vi "Build Async Send Method.vi"(6 "Wiring Spec":T2, 7 "Async AF Library FQN":string, 8 "error in (no error)":errorcluster, 9 "AF Library FQN":string, 10 "References":T1, 11 "Send VI":refnum<vi>) -> (0 "error out":errorcluster)   [LabVIEW 2023, in "Message Maker.lvclass"]
doc: "Build The send vi for the new Async message"
uses:
  Message Maker.lvclass
  Wiring Spec.ctl
  Connector Pane Position.ctl
  Scripting Refs.ctl
  <vilib>/Utility/traverseref.llb/TRef TravTarget.ctl
  <vilib>/Utility/miscctls.llb/LVPointTypeDef.ctl
  Message Maker.lvclass/Message Maker.ctl
  <vilib>/Utility/traverseref.llb/VI Scripting - Traverse.lvlib
  <vilib>/LabVIEW Icon API/LabVIEW Icon API.lvlib
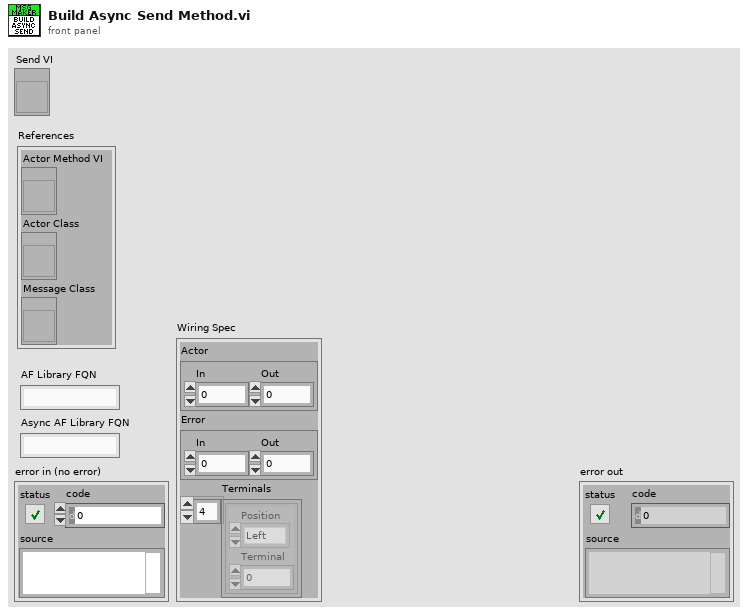
[diagram p1: front panel]
types:
  T1 = typedef "Message Maker.lvclass/Scripting Refs.ctl" = cluster{"Actor Method VI":refnum<vi>, "Actor Class":refnum<vi>, "Message Class":refnum<vi>}
  T2 = typedef "Message Maker.lvclass/Wiring Spec.ctl" = cluster{"Actor":cluster{"In":i32, "Out":i32}, "Error":cluster{"In":i32, "Out":i32}, "Terminals":cluster{"Position":T3, "Terminal":i32}[]}
  T3 = typedef "Message Maker.lvclass/Connector Pane Position.ctl" = enum16{"Left", "Top", "Bottom", "Right"}
  T4 = cluster{"Left":cluster{"Position":i16, "Index":i32}[], "Bottom":cluster{"Position":i16, "Index":i32}[], "Right":cluster{"Position":i16, "Index":i32}[], "Top":cluster{"Position":i16, "Index":i32}[]}
  T5 = enum16{"Replace Classes", "Configure Connector", "Add FP Controls", "Wire Bundle", "Wire Unbundle", "Wire Property Node", "Set Icon and Desc", "Build BD"}
  T6 = typedef "TRef TravTarget.ctl" = enum16{"FP", "BD", "Other"}
  T7 = typedef "LVPointTypeDef.ctl" = cluster{"Horizontal":i16, "Vertical":i16}
  T8 = typedef "LVRectTypeDef.ctl" = cluster{"Left":i16, "Top":i16, "Right":i16, "Bottom":i16}
  T9 = enum16{"Invalid Wire Rule", "Required", "Recommended", "Optional", "Dynamic Dispatch"}[]
  T10 = cluster{cluster{"Position":i16, "Index":i32}[]}[]
  T11 = enum16{"Invalid Wire Rule", "Required", "Recommended", "Optional", "Dynamic Dispatch"}
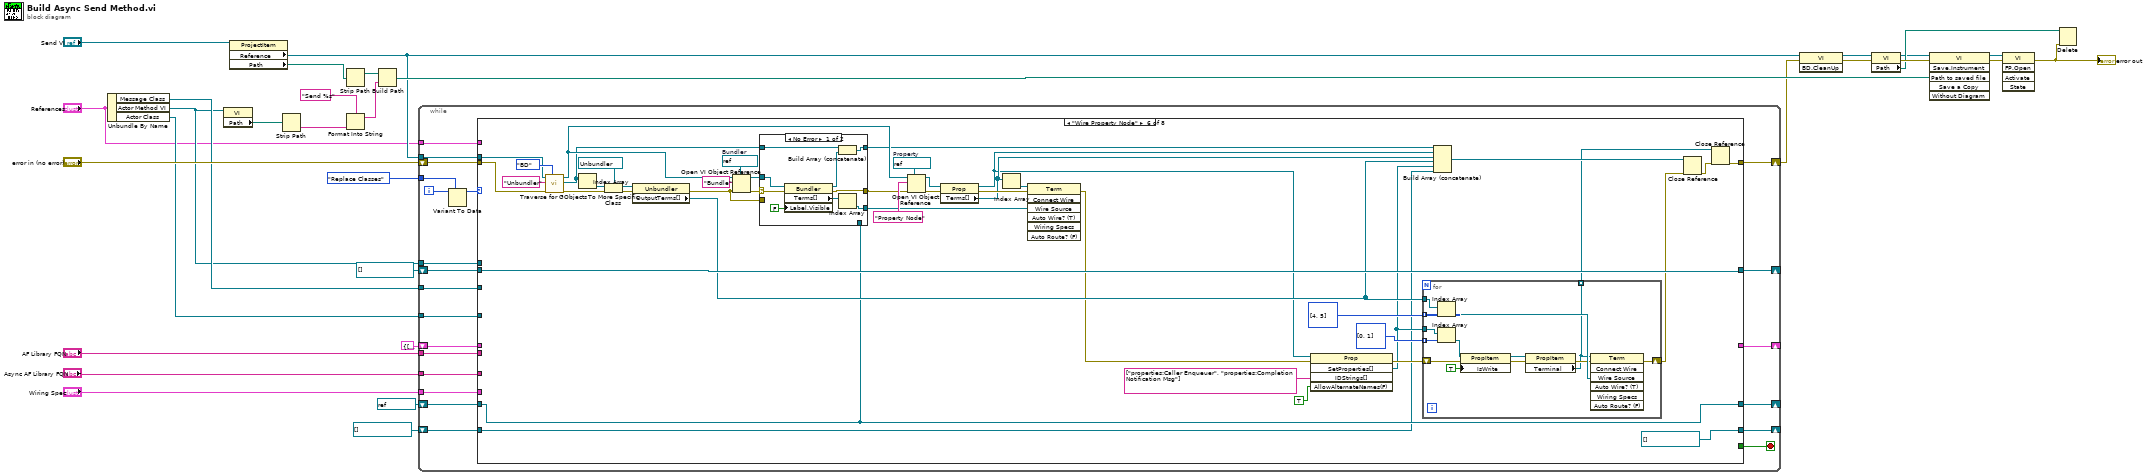
[diagram p0: block diagram]
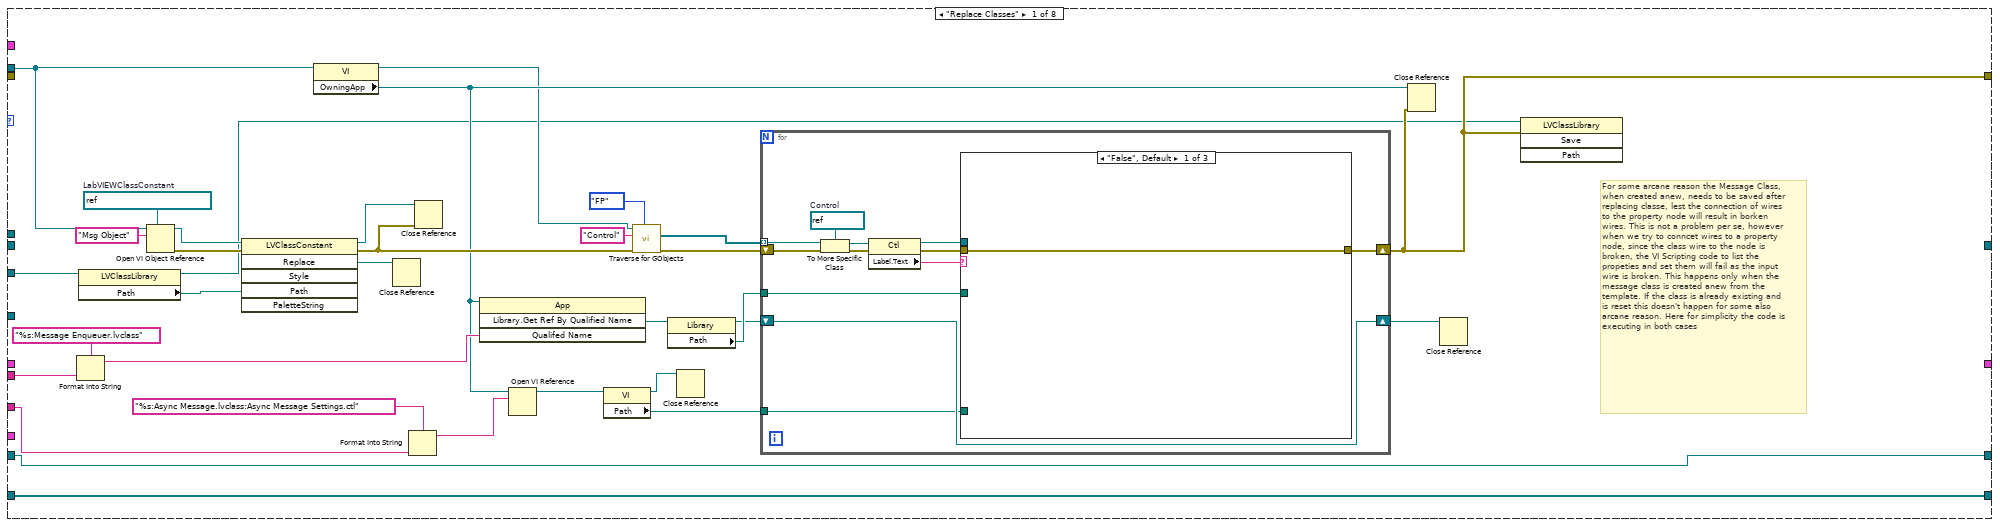
[diagram p2: hidden frame]
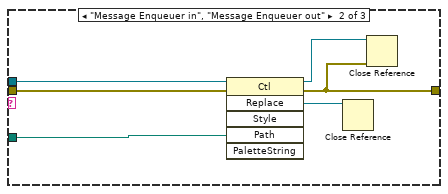
[diagram p3: hidden frame]
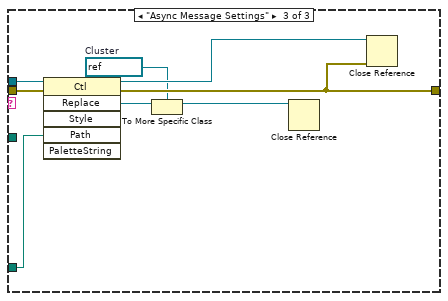
[diagram p4: hidden frame]
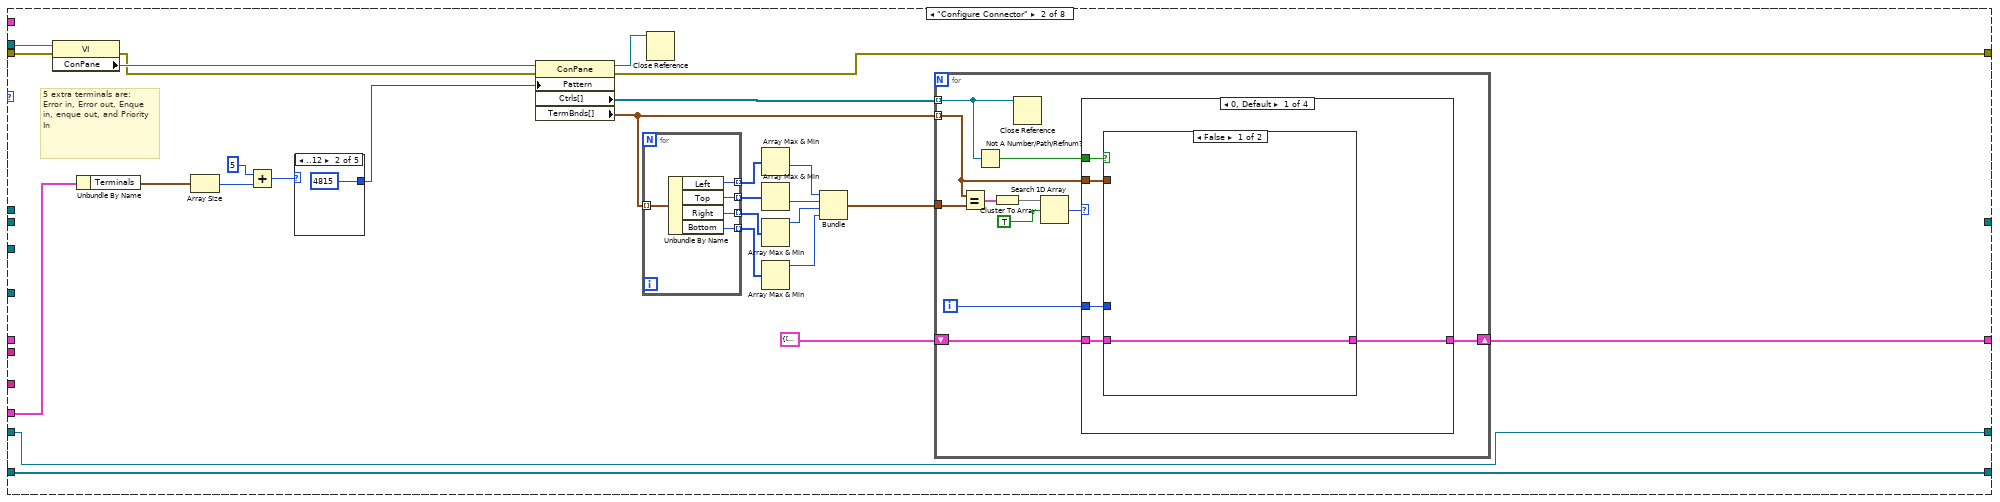
[diagram p5: hidden frame]
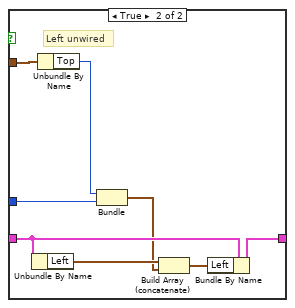
[diagram p6: hidden frame]
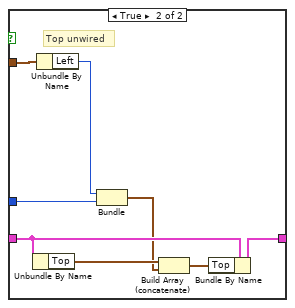
[diagram p8: hidden frame]
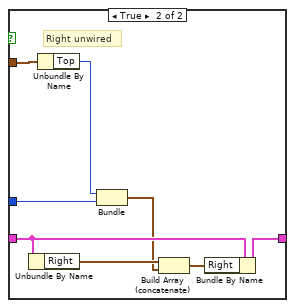
[diagram p10: hidden frame]
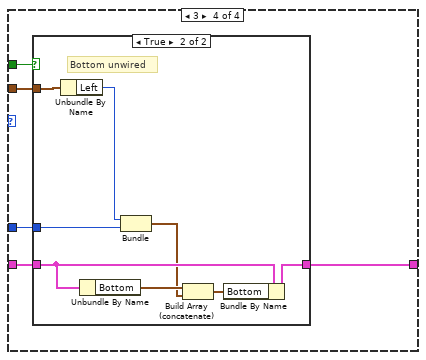
[diagram p11: hidden frame]
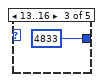
[diagram p14: hidden frame]
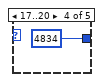
[diagram p15: hidden frame]
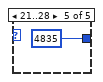
[diagram p16: hidden frame]
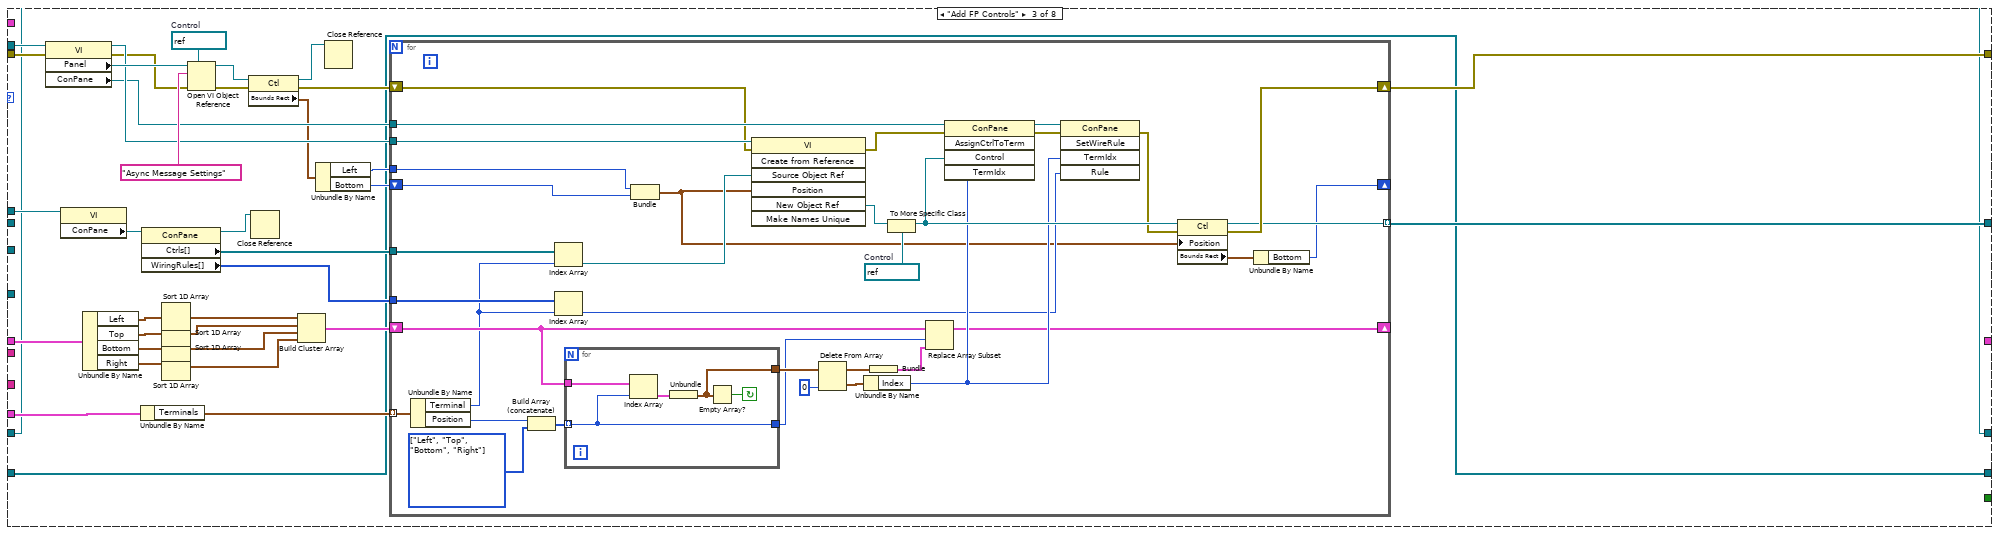
[diagram p17: hidden frame]
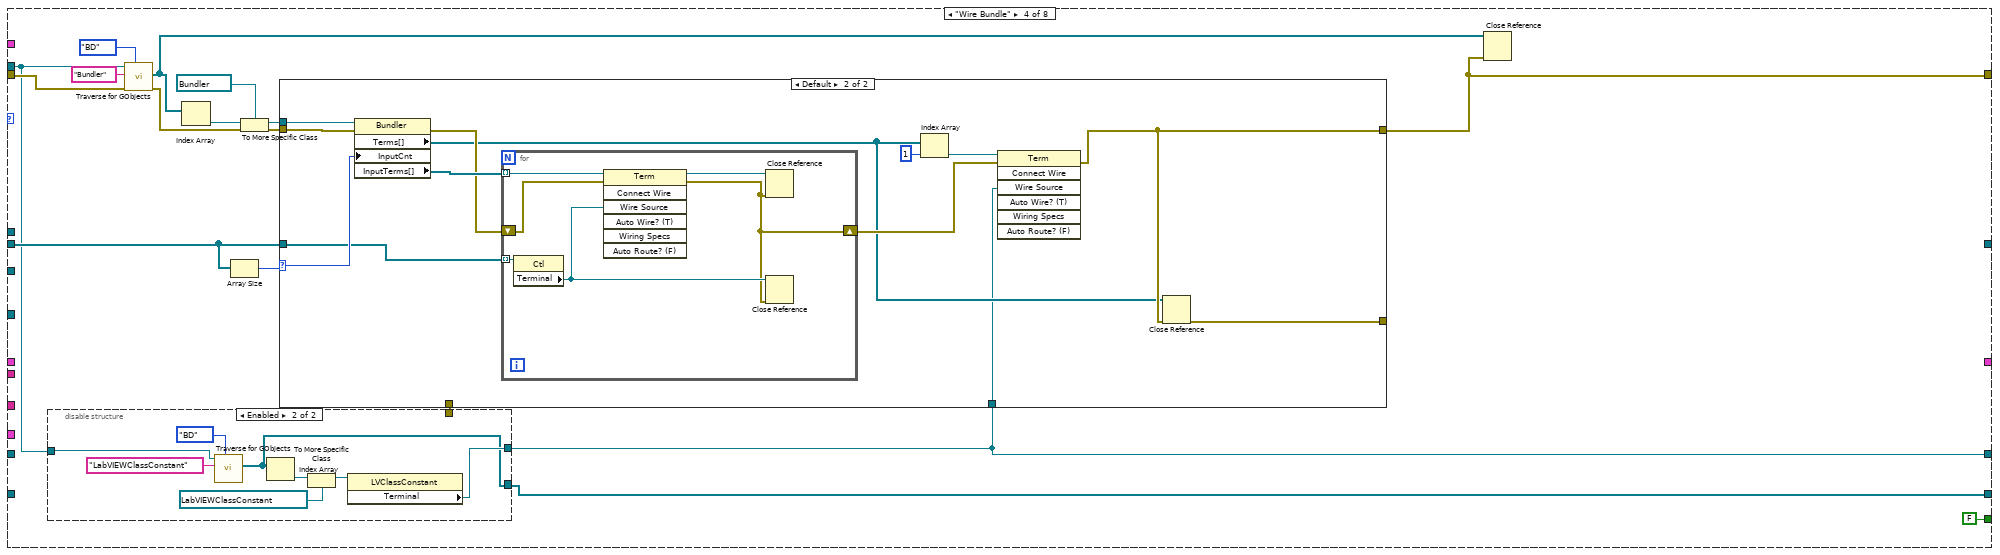
[diagram p18: hidden frame]
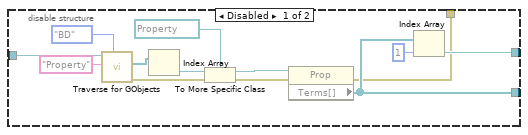
[diagram p19: hidden frame]
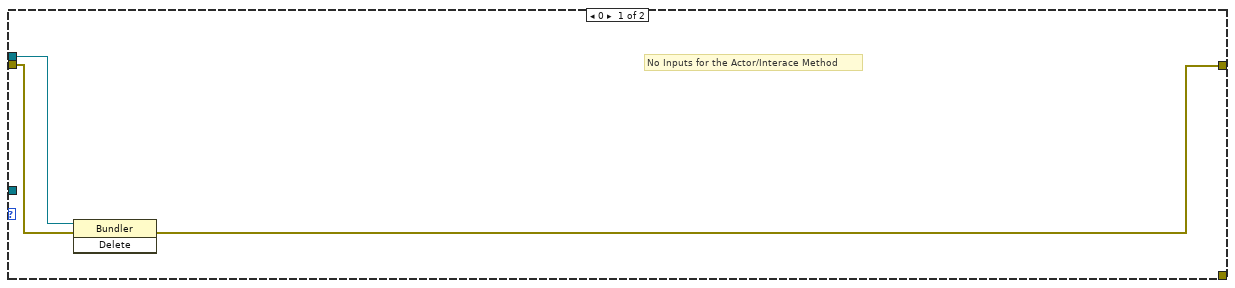
[diagram p20: hidden frame]
diagram:
  n1 = Unbundle By Name("References") -> ("Message Class"=w14:refnum<vi>, "Actor Method VI"=w9:refnum<vi>, "Actor Class"=w13:refnum<vi>)
  n2 = property class="VI"(reference=w9) -> ("Path"=w8:path)  [unwired: 1 in, 2 out]
  n3 = property class="ProjectItem"(reference="Send VI") -> ("Reference"=w22:refnum<vi>, "Path"=w28:path)  [unwired: 1 in, 2 out]
  n4 = Strip Path(path=w8) -> (name=w7:string)  [unwired: 1 out]
  n5 = Strip Path(path=w28) -> (stripped path=w27:path)  [unwired: 1 out]
  n6 = Format Into String(format string="Send %s", w7) -> (resulting string=w26:string)  [unwired: 2 in, 1 out]
  n7 = Build Path(base path=w27, name or relative path=w26) -> (appended path=w25:path)
  n8 = while {
    tunnel: T5."Replace Classes" -> [w53]
    tunnel: "Wiring Spec" -> [w50]
    tunnel: w22 -> [w49]
    tunnel: w9 -> [w48]
    shift-right: [w45] -> w20
    shift-left: "error in (no error)" -> [w46]
    shift-right: [w44] -> _
    shift-left: T4 {"Left"=[], "Bottom"=[], "Right"=[], "Top"=[]} -> [w43]
    shift-right: [w42] -> _
    shift-left: refnum<vi>[] [] -> [w41]
    tunnel: w14 -> [w40]
    tunnel: w13 -> [w39]
    tunnel: "AF Library FQN" -> [w38]
    shift-right: [w37] -> _
    shift-left: refnum<vi>[] [] ("Terms[]") -> [w36]
    tunnel: "Async AF Library FQN" -> [w35]
    tunnel: "References" -> [w34]
    shift-right: [w33] -> _
    shift-left: refnum<vi> refnum ("Terminal") -> [w32]
    i -> [w52]
    stop <- w47 stop-if-true
    n9 = Variant To Data(type=w53, Variant=w52) -> (data=w51:T5)  [unwired: 1 in, 1 out]
    n10 = case shown="\"Wire Property Node\"" w51 {
      tunnel: w50 -> [_ w140 w243 _ _ _ _ _]
      tunnel: w49 -> [w76 w139 w252 w297 w368 w413 w469 w493]
      tunnel: w48 -> [_ _ w245 _ _ _ w470 _]
      tunnel: [_ _ _ FALSE FALSE _ _ TRUE] -> w47
      tunnel: w46 -> [_ w134 w238 w309 w379 w414 w453 w479]
      tunnel: [w56 w132 w235 w298 w370 w422 w451 w487] -> w45
      tunnel: [_ w116 _ _ _ _ _ _] -> w44
      tunnel: w43 -> [_ _ w234 _ _ _ _ _]
      tunnel: [_ _ w222 _ w360 w412 _ _] -> w42
      tunnel: w41 -> [_ _ _ w304 w360 w412 _ _]
      tunnel: w40 -> [w84 _ _ _ _ _ w462 _]
      tunnel: w39 -> [_ _ _ _ _ _ w460 _]
      tunnel: w38 -> [w60 _ _ _ _ _ _ _]
      tunnel: [w62 w115 w218 w296 w363 refnum<vi>[] [] ("References") w450 w516] -> w37
      tunnel: w36 -> [w62 w115 w218 _ w363 w383 w450 w516]
      tunnel: w35 -> [w59 _ _ _ _ _ _ w475]
      tunnel: w34 -> [_ _ _ _ _ _ _ _]
      tunnel: [w54 w114 w217 w293 w353 w384 w449 w471] -> w33
      tunnel: w32 -> [w54 w114 w217 _ w353 w384 w449 w471]
      frame "Replace Classes" {
        w82 = refnum<vi> refnum  # LabVIEWClassConstant
        # "For some arcane reason the Message Class, when created anew, needs to be saved after replacing classe, lest the connection of wires to the property node will result in borken wires. This is not a problem per se, however when we try to conncet wires to a property node, since the class wire to the node is broken, the VI Scripting code to list the propeties and set them will fail as the input wire is broken. This happens only when the message class is created anew from the template. If the class is already existing and is reset this doesn't happen for some also arcane reason. Here for simplicity the code is executing in both cases"
        n11 = Format Into String(format string="%s:Message Enqueuer.lvclass", w60) -> (resulting string=w65:string)  [unwired: 2 in, 1 out]
        n12 = property class="LVClassLibrary"(reference=w84) -> (reference out=w55:refnum<vi>, "Path"=w86:path)  [unwired: 1 in, 1 out]
        n13 = Open VI Object Reference(7:w82, 10:"Msg Object" ("name/order"), 11:w76) -> (0:w83:errorcluster, 3:w58:refnum<vi>)  [unwired: 1 in]
        n14 = invoke class="LVClassConstant" method="Replace"(reference=w58, error in=w83, "Path"=w86) -> (reference out=w81:refnum<vi>, error out=w77:errorcluster, "Replace"=w85:refnum<vi>)  [unwired: 3 in, 3 out]
        n15 = property class="VI"(reference=w76) -> (reference out=w57:refnum<vi>, "OwningApp"=w63:refnum<vi>)  [unwired: 1 in, 1 out]
        n16 = Close Reference(reference=w85) -> ()  [unwired: 1 in, 1 out]
        n17 = Format Into String(format string="%s:Async Message.lvclass:Async Message Settings.ctl", w59) -> (resulting string=w69:string)  [unwired: 2 in, 1 out]
        n18 = Close Reference(reference=w81, error in (no error)=w77) -> ()  [unwired: 1 out]
        n19 = invoke class="App" method="Library.Get Ref By Qualified Name"(reference=w63, "Qualifed Name"=w65) -> ("Library.Get Ref By Qualified Name"=w73:refnum<vi>)  [unwired: 2 in, 3 out]
        n20 = Open VI Reference(application reference (local)=w63, vi path=w69) -> (vi reference=w68:refnum<vi>)  [unwired: 4 in, 1 out]
        n21 = property class="VI"(reference=w68) -> (reference out=w64:refnum<vi>, "Path"=w67:path)  [unwired: 1 in, 1 out]
        n22 = call <vilib>:"Traverse for GObjects.vi"("Traverse Target"=TRef_TravTarget."FP", "error in (no error)"=w77, "Class Name"="Control" ("name/order"), "VI Refnum"=w57) -> ("error out"=w78:errorcluster, "References"=w74:refnum<vi>[])  [unwired: 4 in, 2 out]
        n23 = property class="Library"(reference=w73) -> (reference out=w71:refnum<vi>, "Path"=w72:path)  [unwired: 1 in, 1 out]
        n24 = Close Reference(reference=w64) -> ()  [unwired: 1 in, 1 out]
        n25 = for {
          tunnel: w74 -> [w91] mode=indexing
          tunnel: w72 -> [w97]
          shift-right: [w96] -> w56
          shift-left: w78 -> [w98]
          shift-right: [w95] -> w70
          shift-left: w71 -> [w95]
          tunnel: w67 -> [w87]
          w89 = refnum<vi> refnum  # Control
          n26 = To More Specific Class(target class=w89, reference=w91, error in=w98) -> (specific class reference=w90:refnum<vi>, error out=w92:errorcluster)
          n27 = property class="Ctl"(reference=w90, error in=w92) -> (reference out=w93:refnum<vi>, error out=w94:errorcluster, "Label.Text"=w88:string)
          n28 = case shown="\"False\", Default" w88 {
            tunnel: w97 -> [_ w103 _]
            tunnel: [w99 w102 w111] -> w96
            tunnel: w94 -> [w99 w101 w110]
            tunnel: w93 -> [_ w100 w109]
            tunnel: w87 -> [_ _ w108]
            frame "False", Default {
            }
            frame "Message Enqueuer in", "Message Enqueuer out" {
              n29 = invoke class="Ctl" method="Replace"(reference=w100, error in=w101, "Path"=w103) -> (reference out=w105:refnum<vi>, error out=w102:errorcluster, "Replace"=w104:refnum<vi>)  [unwired: 3 in, 3 out]
              n30 = Close Reference(reference=w104) -> ()  [unwired: 1 in, 1 out]
              n31 = Close Reference(reference=w105, error in (no error)=w102) -> ()  [unwired: 1 out]
            }
            frame "Async Message Settings" {
              w106 = refnum<vi> refnum  # Cluster
              n32 = invoke class="Ctl" method="Replace"(reference=w109, error in=w110, "Path"=w108) -> (reference out=w113:refnum<vi>, error out=w111:errorcluster, "Replace"=w112:refnum<vi>)  [unwired: 3 in, 3 out]
              n33 = To More Specific Class(target class=w106, reference=w112) -> (specific class reference=w107:refnum<vi>)  [unwired: 1 in, 1 out]
              n34 = Close Reference(reference=w107) -> ()  [unwired: 1 in, 1 out]
              n35 = Close Reference(reference=w113, error in (no error)=w111) -> ()  [unwired: 1 out]
            }
          }
        }
        n36 = Close Reference(reference=w63, error in (no error)=w56) -> ()  [unwired: 1 out]
        n37 = Close Reference(reference=w70) -> ()  [unwired: 1 in, 1 out]
        n38 = invoke class="LVClassLibrary" method="Save"(reference=w55, error in=w56) -> ()  [unwired: 2 in, 4 out]
      }
      frame "Configure Connector" {
        # "5 extra terminals are:\nError in, Error out, Enque in, enque out, and Priority In"
        n39 = property class="VI"(reference=w139, error in=w134) -> (error out=w133:errorcluster, "ConPane"=w138:refnum<vi>)  [unwired: 1 out]
        n40 = Unbundle By Name(w140) -> ("Terminals"=w137:cluster{"Position":T3, "Terminal":i32}[])
        n41 = Array Size(array=w137) -> (size(s)=w131:i32)
        n42 = Add(x=5, y=w131) -> (x+y=w129:i32)
        n43 = case shown="..12" w129 {
          tunnel: [_ u32 4815 ("Pattern") u32 4833 ("Pattern") u32 4834 ("Pattern") u32 4835 ("Pattern")] -> w135
          frame Default {
          }
          frame ..12 {
          }
          frame 13..16 {
          }
          frame 17..20 {
          }
          frame 21..28 {
          }
        }
        n44 = property class="ConPane"(reference=w138, error in=w133, "Pattern"=w135) -> (reference out=w136:refnum<vi>, error out=w132:errorcluster, "Ctrls[]"=w122:refnum<vi>[], "TermBnds[]"=w120:T8[])
        n45 = for {
          tunnel: w120 -> [w212] mode=indexing
          tunnel: [w211] -> w128 mode=indexing
          tunnel: [w210] -> w127 mode=indexing
          tunnel: [w209] -> w126 mode=indexing
          tunnel: [w208] -> w125 mode=indexing
          n46 = Unbundle By Name(w212) -> ("Left"=w211:i16, "Top"=w210:i16, "Right"=w209:i16, "Bottom"=w208:i16)
        }
        n47 = Close Reference(reference=w136) -> ()  [unwired: 1 in, 1 out]
        n48 = Array Max & Min(array=w128) -> (min value=w119:i16)  [unwired: 3 out]
        n49 = Array Max & Min(array=w127) -> (min value=w118:i16)  [unwired: 3 out]
        n50 = Array Max & Min(array=w126) -> (max value=w124:i16)  [unwired: 3 out]
        n51 = Array Max & Min(array=w125) -> (max value=w123:i16)  [unwired: 3 out]
        n52 = Bundle(w119, w118, w124, w123) -> (w121:cluster{i16, i16, i16, i16})  [unwired: 1 in]
        n53 = for {
          tunnel: w122 -> [w146] mode=indexing
          tunnel: w121 -> [w151]
          tunnel: w120 -> [w143] mode=indexing
          shift-right: [w142] -> w116
          shift-left: T4 {"Left"=[], "Bottom"=[], "Right"=[], "Top"=[]} -> [w144]
          i -> [w141]
          n54 = Equal?(x=w143, y=w151) -> (x = y?=w150:cluster{bool, bool, bool, bool})
          n55 = Not A Number/Path/Refnum?(number/path/refnum=w146) -> (NaN/Path/Refnum?=w145:bool)
          n56 = Cluster To Array(cluster=w150) -> (array=w149:bool[])
          n57 = Close Reference(reference=w146) -> ()  [unwired: 1 in, 1 out]
          n58 = Search 1D Array(1D array=w149, element=TRUE) -> (index of element=w147:i32)  [unwired: 1 in]
          n59 = case shown="0, Default" w147 {
            tunnel: w145 -> [w156 w170 w184 w198]
            tunnel: w144 -> [w155 w169 w183 w197]
            tunnel: w143 -> [w154 w168 w182 w196]
            tunnel: [w153 w167 w181 w195] -> w142
            tunnel: w141 -> [w152 w166 w180 w194]
            frame 0, Default {
              n60 = case shown="False" w156 {
                tunnel: w155 -> [w157 w164]
                tunnel: w154 -> [_ w165]
                tunnel: [w157 w161] -> w153
                tunnel: w152 -> [_ w162]
                frame False {
                }
                frame True {
                  # "Left unwired"
                  n61 = Unbundle By Name(w164) -> ("Left"=w160:cluster{"Position":i16, "Index":i32}[])
                  n62 = Unbundle By Name(w165) -> ("Top"=w163:i16)
                  n63 = Bundle("Top"=w163, w162) -> (w158:cluster{"Top":i16, i32})  [unwired: 1 in]
                  n64 = Build Array (concatenate)(w160, w158) -> (w159:cluster{"Top":i16, "Index":i32}[])
                  n65 = Bundle By Name(cluster=w164, "Left"=w159) -> (w161:T4)
                }
              }
            }
            frame 1 {
              n66 = case shown="False" w170 {
                tunnel: w169 -> [w171 w178]
                tunnel: w168 -> [_ w179]
                tunnel: [w171 w175] -> w167
                tunnel: w166 -> [_ w176]
                frame False {
                }
                frame True {
                  # "Top unwired"
                  n67 = Unbundle By Name(w178) -> ("Top"=w174:cluster{"Position":i16, "Index":i32}[])
                  n68 = Unbundle By Name(w179) -> ("Left"=w177:i16)
                  n69 = Bundle("Left"=w177, w176) -> (w172:cluster{"Left":i16, i32})  [unwired: 1 in]
                  n70 = Build Array (concatenate)(w174, w172) -> (w173:cluster{"Left":i16, "Index":i32}[])
                  n71 = Bundle By Name(cluster=w178, "Top"=w173) -> (w175:T4)
                }
              }
            }
            frame 2 {
              n72 = case shown="False" w184 {
                tunnel: w183 -> [w185 w192]
                tunnel: w182 -> [_ w193]
                tunnel: [w185 w189] -> w181
                tunnel: w180 -> [_ w190]
                frame False {
                }
                frame True {
                  # "Right unwired"
                  n73 = Unbundle By Name(w192) -> ("Right"=w188:cluster{"Position":i16, "Index":i32}[])
                  n74 = Unbundle By Name(w193) -> ("Top"=w191:i16)
                  n75 = Bundle("Top"=w191, w190) -> (w186:cluster{"Top":i16, i32})  [unwired: 1 in]
                  n76 = Build Array (concatenate)(w188, w186) -> (w187:cluster{"Top":i16, "Index":i32}[])
                  n77 = Bundle By Name(cluster=w192, "Right"=w187) -> (w189:T4)
                }
              }
            }
            frame 3 {
              n78 = case shown="True" w198 {
                tunnel: w197 -> [w199 w206]
                tunnel: w196 -> [_ w207]
                tunnel: [w199 w203] -> w195
                tunnel: w194 -> [_ w204]
                frame False {
                }
                frame True {
                  # "Bottom unwired"
                  n79 = Unbundle By Name(w207) -> ("Left"=w205:i16)
                  n80 = Unbundle By Name(w206) -> ("Bottom"=w202:cluster{"Position":i16, "Index":i32}[])
                  n81 = Bundle("Left"=w205, w204) -> (w200:cluster{"Left":i16, i32})  [unwired: 1 in]
                  n82 = Build Array (concatenate)(w202, w200) -> (w201:cluster{"Left":i16, "Index":i32}[])
                  n83 = Bundle By Name(cluster=w206, "Bottom"=w201) -> (w203:T4)
                }
              }
            }
          }
        }
      }
      frame "Add FP Controls" {
        w251 = refnum<vi> refnum  # Control
        n84 = property class="VI"(reference=w252, error in=w238) -> (reference out=w240:refnum<vi>, error out=w237:errorcluster, "Panel"=w249:refnum<vi>, "ConPane"=w239:refnum<vi>)
        n85 = property class="VI"(reference=w245) -> ("ConPane"=w244:refnum<vi>)  [unwired: 1 in, 2 out]
        n86 = Unbundle By Name(w234) -> ("Left"=w233:cluster{"Position":i16, "Index":i32}[], "Top"=w232:cluster{"Position":i16, "Index":i32}[], "Bottom"=w230:cluster{"Position":i16, "Index":i32}[], "Right"=w231:cluster{"Position":i16, "Index":i32}[])
        n87 = Unbundle By Name(w243) -> ("Terminals"=w241:cluster{"Position":T3, "Terminal":i32}[])
        n88 = property class="ConPane"(reference=w244) -> (reference out=w224:refnum<vi>, "Ctrls[]"=w242:refnum<vi>[], "WiringRules[]"=w225:T9)  [unwired: 1 in, 1 out]
        n89 = Sort 1D Array(array=w233) -> (sorted array=w229:cluster{"Position":i16, "Index":i32}[])
        n90 = Sort 1D Array(array=w232) -> (sorted array=w223:cluster{"Position":i16, "Index":i32}[])
        n91 = Sort 1D Array(array=w230) -> (sorted array=w228:cluster{"Position":i16, "Index":i32}[])
        n92 = Sort 1D Array(array=w231) -> (sorted array=w227:cluster{"Position":i16, "Index":i32}[])
        n93 = Open VI Object Reference(7:w251, 8:w237, 10:"Async Message Settings" ("name/order"), 11:w249) -> (0:w246:errorcluster, 3:w248:refnum<vi>)
        n94 = property class="Ctl"(reference=w248, error in=w246) -> (reference out=w247:refnum<vi>, error out=w236:errorcluster, "Bounds Rect"=w221:T8)
        n95 = Close Reference(reference=w224) -> ()  [unwired: 1 in, 1 out]
        n96 = Build Cluster Array(w229, w223, w228, w227) -> (w226:T10)
        n97 = Unbundle By Name(w221) -> ("Left"=w220:i16, "Bottom"=w219:i16)
        n98 = Close Reference(reference=w247) -> ()  [unwired: 1 in, 1 out]
        n99 = for {
          tunnel: w242 -> [w287]
          tunnel: w241 -> [w279] mode=indexing
          tunnel: w240 -> [w286]
          tunnel: w239 -> [w285]
          shift-right: [w280] -> w235
          shift-left: w236 -> [w282]
          shift-right: [w264] -> _
          shift-left: w226 -> [w272]
          tunnel: w225 -> [w263]
          tunnel: [w260] -> w222 mode=indexing
          tunnel: w220 -> [w254]
          shift-right: [w255] -> _
          shift-left: w219 -> [w253]
          w277 = T3[] [enum."Left", enum."Top", enum."Bottom", enum."Right"] items=["Left", "Top", "Bottom", "Right"] ("appended array")
          w284 = refnum<vi> refnum  # Control
          n100 = Unbundle By Name(w279) -> ("Terminal"=w261:i32, "Position"=w278:T3)
          n101 = Build Array (concatenate)(w278, w277) -> (w276:T3[])
          n102 = Index Array(array=w287, index=w261) -> (element=w258:refnum<vi>)
          n103 = Index Array(array=w263, index=w261) -> (element=w262:T11)
          n104 = for {
            tunnel: w272 -> [w292]
            tunnel: w276 -> [w289] mode=indexing
            tunnel: [w289] -> w270
            tunnel: [w288] -> w275
            stop <- w290 continue-if-true
            n105 = Index Array(array=w292, index=w289) -> (element=w291:cluster{cluster{"Position":i16, "Index":i32}[]})
            n106 = Unbundle(w291) -> (w288:cluster{"Position":i16, "Index":i32}[])
            n107 = Empty Array?(array=w288) -> (empty?=w290:bool)
          }
          n108 = Bundle("Left"=w254, "Bottom"=w253) -> (w257:cluster{"Left":i16, "Bottom":i16})  [unwired: 1 in]
          n109 = invoke class="VI" method="Create from Reference"(reference=w286, error in=w282, "Source Object Ref"=w258, "Position"=w257) -> (error out=w281:errorcluster, "New Object Ref"=w259:refnum<vi>)  [unwired: 3 in, 5 out]
          n110 = Delete From Array(array=w275, index=0) -> (deleted portion=w269:cluster{"Position":i16, "Index":i32}, array with subset deleted=w273:cluster{"Position":i16, "Index":i32}[])  [unwired: 1 in]
          n111 = Unbundle By Name(w269) -> ("Index"=w265:i32)
          n112 = Bundle(w273) -> (w271:cluster{cluster{"Position":i16, "Index":i32}[]})  [unwired: 1 in]
          n113 = To More Specific Class(target class=w284, reference=w259) -> (specific class reference=w283:refnum<vi>)  [unwired: 1 in, 1 out]
          n114 = Replace Array Subset(array=w272, new element=w271, index=w270) -> (w264:T10)
          n115 = invoke class="ConPane" method="AssignCtrlToTerm"(reference=w285, error in=w281, "Control"=w283, "TermIdx"=w265) -> (reference out=w268:refnum<vi>, error out=w267:errorcluster)  [unwired: 1 in, 3 out]
          n116 = invoke class="ConPane" method="SetWireRule"(reference=w268, error in=w267, "TermIdx"=w265, "Rule"=w262) -> (error out=w266:errorcluster)  [unwired: 1 in, 4 out]
          n117 = property class="Ctl"(reference=w283, error in=w266, "Position"=w257) -> (reference out=w260:refnum<vi>, error out=w280:errorcluster, "Bounds Rect"=w256:T8)
          n118 = Unbundle By Name(w256) -> ("Bottom"=w255:i16)
        }
      }
      frame "Wire Bundle" {
        n119 = disable-structure shown="Enabled" {
          disable-tunnel: w297 -> [w322 w324]
          disable-tunnel: [w320 w325] -> w293
          disable-tunnel: [w319 w323] -> w296
          disable-tunnel: [w317 _] -> w295
          frame Disabled {
            n120 = call <vilib>:"Traverse for GObjects.vi"("Traverse Target"=TRef_TravTarget."BD", "Class Name"="Property", "VI Refnum"=w322) -> ("error out"=w314:errorcluster, "References"=w315:refnum<vi>[])  [unwired: 5 in, 2 out]
            n121 = Index Array(array=w315) -> (element=w313:refnum<vi>)  [unwired: 1 in]
            n122 = To More Specific Class(target class=refnum<vi> refnum ("element"), reference=w313, error in=w314) -> (specific class reference=w321:refnum<vi>, error out=w318:errorcluster)
            n123 = property class="Prop"(reference=w321, error in=w318) -> (error out=w317:errorcluster, "Terms[]"=w319:refnum<vi>[])  [unwired: 1 out]
            n124 = Index Array(array=w319, index=1) -> (element=w320:refnum<vi>)
          }
          frame Enabled {
            n125 = call <vilib>:"Traverse for GObjects.vi"("Traverse Target"=TRef_TravTarget."BD", "Class Name"="LabVIEWClassConstant", "VI Refnum"=w324) -> ("References"=w323:refnum<vi>[])  [unwired: 5 in, 3 out]
            n126 = Index Array(array=w323) -> (element=w329:refnum<vi>)  [unwired: 1 in]
            n127 = To More Specific Class(target class=refnum<vi> refnum ("element"), reference=w329) -> (specific class reference=w330:refnum<vi>)  [unwired: 1 in, 1 out]
            n128 = property class="LVClassConstant"(reference=w330) -> ("Terminal"=w325:refnum<vi>)  [unwired: 1 in, 2 out]
          }
        }
        n129 = call <vilib>:"Traverse for GObjects.vi"("Traverse Target"=TRef_TravTarget."BD", "error in (no error)"=w309, "Class Name"="Bundler", "VI Refnum"=w297) -> ("error out"=w301:errorcluster, "References"=w299:refnum<vi>[])  [unwired: 4 in, 2 out]
        n130 = Index Array(array=w299) -> (element=w306:refnum<vi>)  [unwired: 1 in]
        n131 = Array Size(array=w304) -> (size(s)=w303:i32)
        n132 = To More Specific Class(target class=refnum<vi> refnum ("element"), reference=w306, error in=w301) -> (specific class reference=w302:refnum<vi>, error out=w300:errorcluster)
        n133 = case shown="Default" w303 {
          selector: w303 -> [_ w344]
          tunnel: w304 -> [_ w342]
          tunnel: w302 -> [w333 w346]
          tunnel: w300 -> [w332 w345]
          tunnel: [w331 w337] -> w298
          tunnel: w293 -> [_ w335]
          tunnel: [_ w334] -> _
          tunnel: w295 -> [_ _]
          frame 0 {
            # "No Inputs for the Actor/Interace Method"
            n134 = invoke class="Bundler" method="Delete"(reference=w333, error in=w332) -> (error out=w331:errorcluster)  [unwired: 1 in, 2 out]
          }
          frame Default {
            n135 = property class="Bundler"(reference=w346, error in=w345, "InputCnt"=w344) -> (error out=w339:errorcluster, "Terms[]"=w336:refnum<vi>[], "InputTerms[]"=w343:refnum<vi>[])  [unwired: 1 out]
            n136 = for {
              tunnel: w343 -> [w352] mode=indexing
              tunnel: w342 -> [w350] mode=indexing
              shift-right: [w348] -> w340
              shift-left: w339 -> [w347]
              n137 = property class="Ctl"(reference=w350) -> ("Terminal"=w349:refnum<vi>)  [unwired: 1 in, 2 out]
              n138 = invoke class="Term" method="Connect Wire"(reference=w352, error in=w347, "Wire Source"=w349) -> (reference out=w351:refnum<vi>, error out=w348:errorcluster)  [unwired: 4 in, 5 out]
              n139 = Close Reference(reference=w351, error in (no error)=w348) -> ()  [unwired: 1 out]
              n140 = Close Reference(reference=w349, error in (no error)=w348) -> ()  [unwired: 1 out]
            }
            n141 = Index Array(array=w336, index=1) -> (element=w341:refnum<vi>)
            n142 = invoke class="Term" method="Connect Wire"(reference=w341, error in=w340, "Wire Source"=w335) -> (error out=w337:errorcluster)  [unwired: 4 in, 6 out]
            n143 = Close Reference(reference=w336, error in (no error)=w337) -> (error out=w334:errorcluster)
          }
        }
        n144 = Close Reference(reference=w299, error in (no error)=w298) -> ()  [unwired: 1 out]
      }
      frame "Wire Unbundle" {
        n145 = call <vilib>:"Traverse for GObjects.vi"("Traverse Target"=TRef_TravTarget."BD", "error in (no error)"=w379, "Class Name"="Unbundler", "VI Refnum"=w368) -> ("error out"=w373:errorcluster, "References"=w371:refnum<vi>[], "dup VI Refnum"=w359:refnum<vi>)  [unwired: 4 in, 1 out]
        n146 = Index Array(array=w371) -> (element=w376:refnum<vi>)  [unwired: 1 in]
        n147 = To More Specific Class(target class=refnum<vi> refnum ("element"), reference=w376, error in=w373) -> (specific class reference=w374:refnum<vi>, error out=w372:errorcluster)
        n148 = property class="Unbundler"(reference=w374, error in=w372) -> (error out=w358:errorcluster, "Terms[]"=w355:refnum<vi>[])  [unwired: 1 out]
        n149 = Open VI Object Reference(7:refnum<vi> refnum ("element"), 8:w358, 10:"Async Message Settings" ("name/order"), 11:w359) -> (0:w357:errorcluster, 3:w366:refnum<vi>)
        n150 = property class="Ctl"(reference=w366, error in=w357) -> (error out=w356:errorcluster, "Terminal"=w364:refnum<vi>)  [unwired: 1 out]
        n151 = Index Array(array=w355, index=0) -> (element=w361:refnum<vi>)
        n152 = invoke class="Term" method="Connect Wire"(reference=w361, error in=w356, "Wire Source"=w364) -> (error out=w370:errorcluster)  [unwired: 4 in, 6 out]
        n153 = Close Reference(reference=w355, error in (no error)=w370) -> (error out=w365:errorcluster)
        n154 = Close Reference(reference=w371, error in (no error)=w370) -> ()  [unwired: 1 out]
        n155 = Close Reference(reference=w364, error in (no error)=w365) -> ()  [unwired: 1 out]
      }
      frame "Wire Property Node" {
        w397 = refnum<vi> refnum  # Bundler
        w410 = refnum<vi> refnum  # Property
        n156 = call <vilib>:"Traverse for GObjects.vi"("Traverse Target"=TRef_TravTarget."BD", "error in (no error)"=w414, "Class Name"="Unbundler", "VI Refnum"=w413) -> ("error out"=w416:errorcluster, "References"=w381:refnum<vi>[], "dup VI Refnum"=w386:refnum<vi>)  [unwired: 4 in, 1 out]
        n157 = Index Array(array=w381) -> (element=w419:refnum<vi>)  [unwired: 1 in]
        n158 = To More Specific Class(target class=refnum<vi> refnum ("element"), reference=w419, error in=w416) -> (specific class reference=w417:refnum<vi>, error out=w415:errorcluster)
        n159 = property class="Unbundler"(reference=w417, error in=w415) -> (error out=w395:errorcluster, "OutputTerms[]"=w401:refnum<vi>[])  [unwired: 1 out]
        n160 = Open VI Object Reference(7:w397, 8:w395, 10:"Bundle" ("name/order"), 11:w386) -> (0:w399:errorcluster, 3:w398:refnum<vi>)
        n161 = case shown="No Error" w399 {
          selector: w399 -> [w428 _]
          tunnel: w398 -> [w432 _]
          tunnel: [w430 w434] -> w393
          tunnel: [w427 w435] -> w394
          tunnel: w395 -> [_ w435]
          tunnel: w384 -> [_ w434]
          tunnel: w381 -> [w426 w433]
          tunnel: [w424 w433] -> w380
          frame No Error {
            n162 = property class="Bundler"(reference=w432, error in=w428, "Label.Visible"=FALSE) -> (reference out=w425:refnum<vi>, error out=w427:errorcluster, "Terms[]"=w431:refnum<vi>[])
            n163 = Build Array (concatenate)(w426, w425) -> (w424:refnum<vi>[])
            n164 = Index Array(array=w431) -> (element=w430:refnum<vi>)  [unwired: 1 in]
          }
          frame Error {
          }
        }
        n165 = Open VI Object Reference(7:w410, 8:w394, 10:"Property Node" ("name/order"), 11:w386) -> (0:w406:errorcluster, 3:w391:refnum<vi>)
        n166 = property class="Prop"(reference=w391, error in=w406) -> (reference out=w385:refnum<vi>, error out=w405:errorcluster, "Terms[]"=w402:refnum<vi>[])
        n167 = Index Array(array=w402) -> (element=w407:refnum<vi>)  [unwired: 1 in]
        n168 = invoke class="Term" method="Connect Wire"(reference=w407, error in=w405, "Wire Source"=w393) -> (error out=w387:errorcluster)  [unwired: 4 in, 6 out]
        n169 = invoke class="Prop" method="SetProperties[]"(reference=w385, error in=w387, "IDStrings[]"=string[] ["properties:Caller Enqueuer", "properties:Completion Notification Msg"] ("ID Strings[]"), "AllowAlternateNames(F)"=TRUE ("Allow Alternate Names? (F)")) -> (error out=w392:errorcluster, "SetProperties[]"=w389:refnum<vi>[])  [unwired: 1 in, 3 out]
        n170 = for {
          tunnel: i32[] [4, 5] -> [w447] mode=indexing
          tunnel: i32[] [0, 1] -> [w446] mode=indexing
          tunnel: w401 -> [w448]
          tunnel: w389 -> [w445]
          shift-right: [w442] -> w404
          shift-left: w392 -> [w437]
          tunnel: [w441] -> w400 mode=indexing
          n171 = Index Array(array=w448, index=w447) -> (element=w444:refnum<vi>)
          n172 = Index Array(array=w445, index=w446) -> (element=w440:refnum<vi>)
          n173 = property class="PropItem"(reference=w440, error in=w437, "IsWrite"=TRUE ("Is Write")) -> (reference out=w438:refnum<vi>, error out=w436:errorcluster)
          n174 = property class="PropItem"(reference=w438, error in=w436) -> (error out=w443:errorcluster, "Terminal"=w441:refnum<vi>)  [unwired: 1 out]
          n175 = invoke class="Term" method="Connect Wire"(reference=w441, error in=w443, "Wire Source"=w444) -> (error out=w442:errorcluster)  [unwired: 4 in, 6 out]
        }
        n176 = Build Array (concatenate)(w380, w385, w402, w401, w389, w383) -> (w403:refnum<vi>[])
        n177 = Close Reference(reference=w403, error in (no error)=w404) -> (error out=w423:errorcluster)
        n178 = Close Reference(reference=w400, error in (no error)=w423) -> (error out=w422:errorcluster)
      }
      frame "Set Icon and Desc" {
        n179 = property class="LVClassLibrary"(reference=w462) -> ("QualifiedName"=w461:string)  [unwired: 1 in, 2 out]
        n180 = property class="LVClassLibrary"(reference=w460) -> ("QualifiedName"=w456:string)  [unwired: 1 in, 2 out]
        n181 = call <vilib>:"Get VI Icon.vi"("error in (no error)"=w453, "VI Refnum in"=w470) -> ("error out"=w467:errorcluster, "Icon"=w468:refnum<class "Icon.lvclass">, "VI Refnum out"=w466:refnum<vi>)  [unwired: 7 in]
        n182 = call <vilib>:"Set VI Icon.vi"("error in (no error)"=w467, "Icon"=w468, "VI Refnum in"=w469) -> ("error out"=w452:errorcluster, "VI Refnum out"=w464:refnum<vi>)  [unwired: 7 in]
        n183 = String Length(string=w456) -> (length=w459:i32)
        n184 = property class="VI"(reference=w466) -> ("Name"=w458:string, "Description"=w454:string)  [unwired: 1 in, 2 out]
        n185 = Increment(x=w459) -> (x+1=w457:i32)
        n186 = String Subset(string=w458, offset (0)=w457) -> (substring=w455:string)  [unwired: 1 in]
        n187 = Format Into String(format string="Sends the <b>%s</b> Async Message.\n\nThis message will call <b>%s</b> on the <b>%s</b> Async Method Actor.\n\n<b>%s Description</b>\n%s", w461, w455, w456, w455, w454) -> (resulting string=w463:string)  [unwired: 2 in, 1 out]
        n188 = property class="VI"(reference=w464, error in=w452, "Description"=w463) -> (error out=w451:errorcluster)  [unwired: 1 out]
      }
      frame "Build BD" {
        w502 = refnum<vi> refnum  # Property
        w519 = refnum<vi> refnum  # SubVI
        # "#todo make compatible with ppl"
        n189 = property class="VI"(reference=w493, error in=w479) -> (reference out=w480:refnum<vi>, error out=w473:errorcluster, "OwningApp"=w515:refnum<vi>)
        n190 = Format Into String(format string="%s:Async Message.lvclass:Send Async Message.vi", error in=w473, w475) -> (resulting string=w474:string, error out=w472:errorcluster)  [unwired: 1 in]
        n191 = call <vilib>:"Traverse for GObjects.vi"("Traverse Target"=TRef_TravTarget."BD", "error in (no error)"=w479, "Class Name"="Unbundler", "VI Refnum"=w493) -> ("error out"=w508:errorcluster, "References"=w509:refnum<vi>[])  [unwired: 4 in, 2 out]
        n192 = Index Array(array=w509) -> (element=w507:refnum<vi>)  [unwired: 1 in]
        n193 = Open VI Reference(application reference (local)=w515, vi path=w474, error in (no error)=w472) -> (vi reference=w492:refnum<vi>, error out=w514:errorcluster)  [unwired: 3 in]
        n194 = To More Specific Class(target class=refnum<vi> refnum ("element"), reference=w507, error in=w508) -> (specific class reference=w511:refnum<vi>, error out=w510:errorcluster)
        n195 = property class="VI"(reference=w492, error in=w514) -> (reference out=w488:refnum<vi>, error out=w500:errorcluster, "Path"=w513:path)
        n196 = property class="Unbundler"(reference=w511, error in=w510) -> (error out=w477:errorcluster, "OutputTerms[]"=w481:refnum<vi>[])  [unwired: 1 out]
        n197 = Close Reference(reference=w488) -> ()  [unwired: 1 in, 1 out]
        n198 = New VI Object(vi object class=w519, owner refnum=w480, position/next to=T7 {"Horizontal"=0, "Vertical"=0} ("location"), 6:w513, 8:w500) -> (object refnum=w490:refnum<vi>, 0:w517:errorcluster)  [unwired: 3 in]
        n199 = Index Array(array=w481) -> (element #1=w497:refnum<vi>, element #2=w495:refnum<vi>, element #3=w496:refnum<vi>, element #4=w498:refnum<vi>)  [unwired: 4 in]
        n200 = Open VI Object Reference(7:w502, 8:w500, 10:"Property Node" ("name/order"), 11:w480) -> (0:w503:errorcluster, 3:w485:refnum<vi>)
        n201 = property class="SubVI"(reference=w490, error in=w517) -> (error out=w518:errorcluster, "Terms[]"=w489:refnum<vi>[])  [unwired: 1 out]
        n202 = property class="Prop"(reference=w485, error in=w503) -> ("Terms[]"=w491:refnum<vi>[])  [unwired: 2 out]
        n203 = Merge Errors(w518, w477) -> (w478:errorcluster)
        n204 = Index Array(array=w491, index #1=3 ("index"), index #2=1 ("index")) -> (element #1=w499:refnum<vi>, element #2=w494:refnum<vi>)
        n205 = for {
          tunnel: w489 -> [w530] mode=indexing
          tunnel: w493 -> [w529]
          shift-right: [w528] -> w487
          shift-left: w478 -> [w527]
          tunnel: w499 -> [w526]
          tunnel: w498 -> [w525]
          tunnel: w497 -> [w524]
          tunnel: w496 -> [w523]
          tunnel: w495 -> [w522]
          tunnel: w494 -> [w521]
          i -> [w531]
          n206 = case shown="2" w531 {
            tunnel: w530 -> [w541 w551 w561 w565 w569 w573 w577 w581 w585 w595 _]
            tunnel: w529 -> [w540 w550 w560 _ _ _ _ _ _ w594 _]
            tunnel: [w532 w542 w552 w563 w567 w571 w575 w579 w584 w586 w596] -> w528
            tunnel: w527 -> [w535 w545 w555 w564 w568 w572 w576 w580 w583 w589 w596]
            tunnel: w526 -> [_ _ _ _ _ _ _ w578 _ _ _]
            tunnel: w525 -> [_ _ _ _ w566 _ _ _ _ _ _]
            tunnel: w524 -> [_ _ _ _ _ _ w574 _ _ _ _]
            tunnel: w523 -> [_ _ _ w562 _ _ _ _ _ _ _]
            tunnel: w522 -> [_ _ _ _ _ w570 _ _ _ _ _]
            tunnel: w521 -> [_ _ _ _ _ _ _ _ w582 _ _]
            frame 0 {
              w538 = refnum<vi> refnum  # Control
              n207 = Open VI Object Reference(7:w538, 8:w535, 10:"error out" ("name/order"), 11:w540) -> (0:w534:errorcluster, 3:w537:refnum<vi>)
              n208 = property class="Ctl"(reference=w537, error in=w534) -> (error out=w533:errorcluster, "Terminal"=w536:refnum<vi>)  [unwired: 1 out]
              n209 = invoke class="Term" method="Connect Wire"(reference=w541, error in=w533, "Wire Source"=w536) -> (error out=w532:errorcluster)  [unwired: 4 in, 6 out]
            }
            frame 2 {
              w548 = refnum<vi> refnum  # Control
              n210 = Open VI Object Reference(7:w548, 8:w545, 10:"GUID" ("name/order"), 11:w550) -> (0:w544:errorcluster, 3:w547:refnum<vi>)
              n211 = property class="Ctl"(reference=w547, error in=w544) -> (error out=w543:errorcluster, "Terminal"=w546:refnum<vi>)  [unwired: 1 out]
              n212 = invoke class="Term" method="Connect Wire"(reference=w551, error in=w543, "Wire Source"=w546) -> (error out=w542:errorcluster)  [unwired: 4 in, 6 out]
            }
            frame 3 {
              w558 = refnum<vi> refnum  # Control
              n213 = Open VI Object Reference(7:w558, 8:w555, 10:"Message Enqueuer out" ("name/order"), 11:w560) -> (0:w554:errorcluster, 3:w557:refnum<vi>)
              n214 = property class="Ctl"(reference=w557, error in=w554) -> (error out=w553:errorcluster, "Terminal"=w556:refnum<vi>)  [unwired: 1 out]
              n215 = invoke class="Term" method="Connect Wire"(reference=w561, error in=w553, "Wire Source"=w556) -> (error out=w552:errorcluster)  [unwired: 4 in, 6 out]
            }
            frame 4 {
              n216 = invoke class="Term" method="Connect Wire"(reference=w565, error in=w564, "Wire Source"=w562) -> (error out=w563:errorcluster)  [unwired: 4 in, 6 out]
            }
            frame 5 {
              n217 = invoke class="Term" method="Connect Wire"(reference=w569, error in=w568, "Wire Source"=w566) -> (error out=w567:errorcluster)  [unwired: 4 in, 6 out]
            }
            frame 6 {
              n218 = invoke class="Term" method="Connect Wire"(reference=w573, error in=w572, "Wire Source"=w570) -> (error out=w571:errorcluster)  [unwired: 4 in, 6 out]
            }
            frame 7 {
              n219 = invoke class="Term" method="Connect Wire"(reference=w577, error in=w576, "Wire Source"=w574) -> (error out=w575:errorcluster)  [unwired: 4 in, 6 out]
            }
            frame 8 {
              n220 = invoke class="Term" method="Connect Wire"(reference=w581, error in=w580, "Wire Source"=w578) -> (error out=w579:errorcluster)  [unwired: 4 in, 6 out]
            }
            frame 10 {
              n221 = invoke class="Term" method="Connect Wire"(reference=w585, error in=w583, "Wire Source"=w582) -> (error out=w584:errorcluster)  [unwired: 4 in, 6 out]
            }
            frame 11 {
              w592 = refnum<vi> refnum  # Control
              n222 = Open VI Object Reference(7:w592, 8:w589, 10:"Message Enqueuer in" ("name/order"), 11:w594) -> (0:w588:errorcluster, 3:w591:refnum<vi>)
              n223 = property class="Ctl"(reference=w591, error in=w588) -> (error out=w587:errorcluster, "Terminal"=w590:refnum<vi>)  [unwired: 1 out]
              n224 = invoke class="Term" method="Connect Wire"(reference=w595, error in=w587, "Wire Source"=w590) -> (error out=w586:errorcluster)  [unwired: 4 in, 6 out]
            }
            frame Default {
            }
          }
        }
        n225 = Build Array (concatenate)(w485, w491, w490, w489) -> (w486:refnum<vi>[])
        n226 = Build Array (concatenate)(w486, w481) -> (w482:refnum<vi>[])
        n227 = Close Reference(reference=w482, error in (no error)=w487) -> ()  [unwired: 1 out]
      }
    }
  }
  n228 = invoke class="VI" method="BD.CleanUp"(reference=w22, error in=w20) -> (reference out=w29:refnum<vi>, error out=w16:errorcluster)  [unwired: 1 in, 1 out]
  n229 = property class="VI"(reference=w29, error in=w16) -> (reference out=w6:refnum<vi>, error out=w17:errorcluster, "Path"=w15:path)
  n230 = invoke class="VI" method="Save.Instrument"(reference=w6, error in=w17, "Path to saved file"=w25) -> (reference out=w12:refnum<vi>, error out=w10:errorcluster)  [unwired: 3 in, 4 out]
  n231 = invoke class="VI" method="FP.Open"(reference=w12, error in=w10) -> (error out=w11:errorcluster)  [unwired: 3 in, 4 out]
  "error out" <- w11
  n232 = Delete(path (use dialog)=w15, error in=w11) -> ()  [unwired: 3 in, 3 out]
